vi "Read Sweep Configuration File.vi"(8 "error in (no error)":errorcluster, 10 "Path":path, 11 "SweepControl in":refnum<class "Sweep Control.lvclass">) -> (0 "error out":errorcluster, 2 "Data":variant, 3 "SweepControl out":refnum<class "Sweep Control.lvclass">)   [LabVIEW 2019, in "Sweep Control.lvclass"]
uses:
  Sweep Control.lvclass
  Typedefs/Enum - Experiments.ctl
  Typedefs/Continuous B Sweep JSON--Cluster.ctl
  Typedefs/Enum - Priority.ctl
  Typedefs/Enum - Action.ctl
  Typedefs/Cluster - ScanControl.ctl
  Typedefs/ScanControl.ctl
  Typedefs/Cluster - ScanParamters.ctl
  Typedefs/ScanParamters.ctl
  Typedefs/Sweep Control JSON--Cluster.ctl
  <userlib>/LevyLab/Transport/Control Experiment/Typedefs/Wiring Description--cluster.ctl
  <userlib>/LevyLab/Transport/Control Experiment/Control Experiment.lvclass
  <userlib>/LevyLab/Transport/Control Experiment/Typedefs/Experiment Description--cluster.ctl
  <userlib>/LevyLab/Transport/Transport/Typedefs/Lockin_Sweep JSON--Cluster.ctl
  <userlib>/LevyLab/Transport/Transport/Transport.lvclass
  <userlib>/LevyLab/Lockin-Multichannel/Instrument.DAQ/Typedefs/REF.Channel--Cluster--Array.ctl
  <userlib>/LevyLab/Lockin-Multichannel/Instrument.DAQ/Instrument.DAQ.lvclass
  <userlib>/LevyLab/Lockin-Multichannel/Instrument.DAQ/Typedefs/AO.Channel--Cluster--Array.ctl
  <userlib>/LevyLab/Transport/Control Experiment/Typedefs/Instruments--cluster.ctl
  <userlib>/LevyLab/Krohn Hite 7008/KH7008/typedefs/Filter--Enum.ctl
  <userlib>/LevyLab/Krohn Hite 7008/KH7008/KH7008.lvlib
  <userlib>/LevyLab/Krohn Hite 7008/KH7008/typedefs/couple--Enum.ctl
  <userlib>/LevyLab/Krohn Hite 7008/KH7008/typedefs/shunt--enum.ctl
  <userlib>/LevyLab/Krohn Hite 7008/KH7008/typedefs/Input--Enum.ctl
  <userlib>/LevyLab/Krohn Hite 7008/KH7008/typedefs/gain--enum.ctl
  <userlib>/LevyLab/Krohn Hite 7008/KH7008/typedefs/channel--numeric.ctl
  <userlib>/LevyLab/Krohn Hite 7008/KH7008/typedefs/channelProperties--Cluster.ctl
  <userlib>/LevyLab/Krohn Hite 7008/KH7008/typedefs/allChannelProperties--Array.ctl
  <userlib>/LevyLab/Lockin-Multichannel/Instrument.DAQ/Typedefs/REF.Channel--Cluster.ctl
  <userlib>/LevyLab/Lockin-Multichannel/Instrument.DAQ/Typedefs/AO.Channel.Function--Enum.ctl
  <userlib>/LevyLab/Lockin-Multichannel/Instrument.DAQ/Typedefs/AO.Channel--Cluster.ctl
  <userlib>/LevyLab/Transport/Control Experiment/Typedefs/Instrument Types--enum.ctl
  88356f33-0b26-47ad-bb5b-a6bd6fb0bfd5.vi
  cc7c3cdd-3319-44b7-ab3c-1b04586ceafc.vi
  36e136b2-e9ff-439f-9429-e3ffdab4ccf7.vi
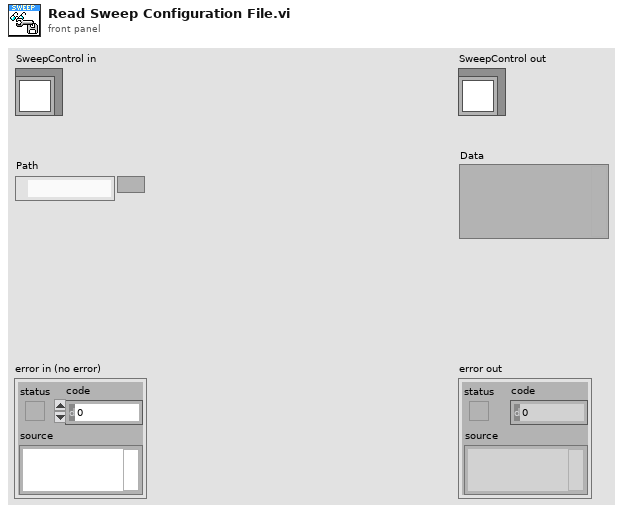
[diagram p1: front panel]
types:
  T1 = typedef "Transport.lvclass/Lockin_Sweep JSON--Cluster.ctl" = cluster{"initialWaitTime":dbl, "sweepTime":dbl, "Return to Start":bool, "sweepChannels":cluster{"Enable?":bool, "Channel":u16, "Start":dbl, "End":dbl, "Pattern":enum16{"Ramp /", "Ramp /\\", "Smooth Ramp _/", "Smooth Ramp _/\\_", "Table"}, "Table":dbl[]}[], "sweepTables":cluster{"Ch":i32, "Table":dbl[]}[]}
  T2 = typedef "Sweep Control.lvclass/Continuous B Sweep JSON--Cluster.ctl" = cluster{"Continuous B Sweep":cluster{"Experiment":T3, "B field values":dbl[]}, "Experiment Description":T4, "Wiring Configuration":T7, "Lockin":cluster{"AOconfig":T8, "REFconfig":T11}, "Krohn Hite":cluster{"Channel Setting":T13}}
  T3 = typedef "Sweep Control.lvclass/Enum - Experiments.ctl" = enum16{"LockinTime", "LockinSweep", "LockinDelayLine"}
  T4 = typedef "Control Experiment.lvclass/Experiment Description--cluster.ctl" = cluster{"User":string, "Device":string, "Device Path":path, "Device Description":string, "Experiment Path":path, "Experiment Description":string, "Instrument":string, "Instruments":T5[], "Sweep":cluster{"key":string, "value":variant}[]}
  T5 = typedef "Control Experiment.lvclass/Instruments--cluster.ctl" = cluster{"class path":path, "Address":string, "Type":T6}
  T6 = typedef "Control Experiment.lvclass/Instrument Types--enum.ctl" = enum16{"DAQ", "Amplifier", "Temperature", "Magnet", "Rotator", "Level", "Capacitance", "Delay Line", "Strain Cell", "VNA", "Source"}
  T7 = typedef "Control Experiment.lvclass/Wiring Description--cluster.ctl" = cluster{"Lockin Ch":i32[], "KH":cluster{"Electrodes":string[], "Labels":string[]}, "not KH":cluster{"Electrodes":string[], "Labels":string[]}}
  T8 = typedef "Instrument.Lockin.lvlib/Instrument.DAQ.lvclass/AO.Channel--Cluster--Array.ctl" = T9[]
  T9 = typedef "Instrument.Lockin.lvlib/Instrument.DAQ.lvclass/AO.Channel--Cluster.ctl" = cluster{"Enable?":bool, "Channel":i32, "Amplitude":dbl, "Offset":dbl, "Frequency":dbl, "Phase":dbl, "Function":T10, "Sweeping?":bool, "Limit AC":bool, "Limit DC?":bool, "Duty Cycle":bool}
  T10 = typedef "Instrument.Lockin.lvlib/Instrument.DAQ.lvclass/AO.Channel.Function--Enum.ctl" = enum16{"sine", "square", "triangle", "saw"}
  T11 = typedef "Instrument.Lockin.lvlib/Instrument.DAQ.lvclass/REF.Channel--Cluster--Array.ctl" = T12[]
  T12 = typedef "Instrument.Lockin.lvlib/Instrument.DAQ.lvclass/REF.Channel--Cluster.ctl" = cluster{"Enable?":bool, "Channel":i32, "Frequency":dbl, "Phase":dbl, "TC":dbl, "Roll-Off":i32}
  T13 = typedef "KH7008.lvlib/allChannelProperties--Array.ctl" = T14[]
  T14 = typedef "KH7008.lvlib/channelProperties--Cluster.ctl" = cluster{"channel":T15, "gain":T16, "input":T17, "shunt":T18, "couple":T19, "filter":T20}
  T15 = typedef "KH7008.lvlib/channel--numeric.ctl" = u16
  T16 = typedef "KH7008.lvlib/gain--enum.ctl" = enum16{"1", "10", "100", "1000"}
  T17 = typedef "KH7008.lvlib/Input--Enum.ctl" = enum16{"OFF", "SE+", "SE-", "DIFF"}
  T18 = typedef "KH7008.lvlib/shunt--enum.ctl" = enum16{"Open", "50", "500", "5k", "50k", "10M"}
  T19 = typedef "KH7008.lvlib/couple--Enum.ctl" = enum16{"AC", "DC"}
  T20 = typedef "KH7008.lvlib/Filter--Enum.ctl" = enum16{"OFF", "ON"}
  T21 = typedef "Sweep Control.lvclass/Sweep Control JSON--Cluster.ctl" = cluster{"Experiment":T3, "Repeat Experiment":i32, "Scan control":T22, "Scan parameters":T26}
  T22 = typedef "Sweep Control.lvclass/ScanControl.ctl" = T23[]
  T23 = typedef "Sweep Control.lvclass/Cluster - ScanControl.ctl" = cluster{"Priority":T24, "Scan name":T25}
  T24 = typedef "Sweep Control.lvclass/Enum - Priority.ctl" = enum16{"Priority 0", "Priority 1", "Priority 2", "Priority 3", "Priority 4", "Priority 5"}
  T25 = typedef "Sweep Control.lvclass/Enum - Action.ctl" = enum16{"OFF", "time", "Lockin Amplitude", "Lockin Frequency", "Lockin Bias", "Delay", "Strain", "DAQ Bias", "Magnet Field", "Temperature", "MW f1", "MW f2", "MW Amplitude1", "MW Amplitude2"}
  T26 = typedef "Sweep Control.lvclass/ScanParamters.ctl" = T27[]
  T27 = typedef "Sweep Control.lvclass/Cluster - ScanParamters.ctl" = cluster{"Start":dbl, "End":dbl, "Step":dbl, "Rate":dbl, "Waveform type":enum16{"linear", "triangle", "power"}, "wait (ms or K)":dbl, "Address":string, "channel":i32}
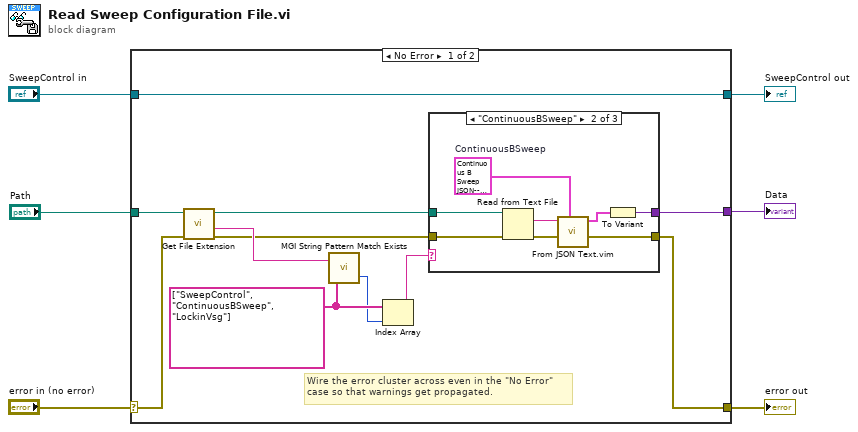
[diagram p0: block diagram]
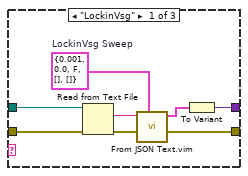
[diagram p2: hidden frame]
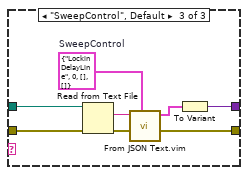
[diagram p3: hidden frame]
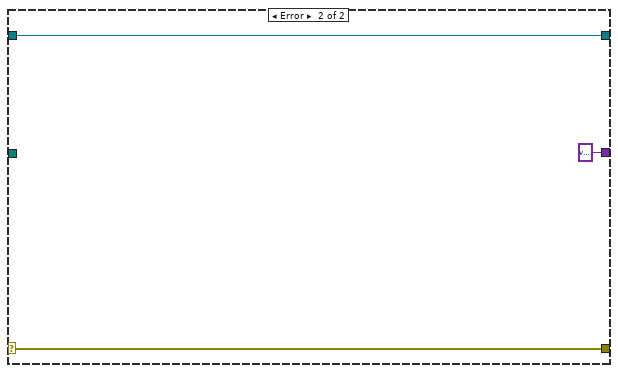
[diagram p4: hidden frame]
diagram:
  n1 = case shown="No Error" "error in (no error)" {
    selector: "error in (no error)" -> [w8 w44]
    tunnel: [w7 w44] -> w5
    tunnel: [w17 w43] -> w3
    tunnel: "SweepControl in" -> [w17 w43]
    tunnel: "Path" -> [w16 _]
    tunnel: [w9 variant ("Variant")] -> w1
    frame No Error {
      w14 = string[] ["SweepControl", "ContinuousBSweep", "LockinVsg"] ("Patterns to Try")
      # "Wire the error cluster across even in the \"No Error\"\ncase so that warnings get propagated."
      n2 = call <vilib>:"Get File Extension.vi"("error in (no error)"=w8, "file"=w16) -> ("error out"=w11:errorcluster, "filename without extension"=w13:string, "dup file"=w10:path)  [unwired: 5 in, 2 out]
      n3 = call <userlib>:"MGI String Pattern Match Exists.vi"("Patterns to Try"=w14, "String"=w13) -> ("Index of First Pattern Matched"=w12:i32)  [unwired: 1 out]
      n4 = Index Array(array=w14, index=w12) -> (element=w15:string)
      n5 = case shown="\"ContinuousBSweep\"" w15 {
        tunnel: w11 -> [w25 w33 w41]
        tunnel: w10 -> [w24 w32 w40]
        tunnel: [w19 w26 w35] -> w9
        tunnel: [w20 w28 w36] -> w7
        frame "LockinVsg" {
          w22 = T1 {"initialWaitTime"=0.001, "sweepTime"=0.0, "Return to Start"=FALSE, "sweepChannels"=[], "sweepTables"=[]}  # LockinVsg Sweep
          n6 = Read from Text File(file (use dialog)=w24, error in=w25) -> (text=w18:string, error out=w21:errorcluster)  [unwired: 2 in, 2 out]
          n7 = call "From JSON Text.vim"("Data Type and Default Value"=w22, "error in (no error)"=w21, "JSON"=w18) -> ("error out"=w20:errorcluster, "Data out"=w23:T1)  [unwired: 7 in]
          n8 = To Variant(anything=w23) -> (Variant=w19:variant)
        }
        frame "ContinuousBSweep" {
          w31 = T2 {"Continuous B Sweep"={"Experiment"=enum."LockinDelayLine", "B field values"=[]}, "Experiment Description"={"User"="", "Device"="", "Device Path"=path "", "Device Description"="", "Experiment Path"=path "", "Experiment Description"="", "Instrument"="", "Instruments"=[], "Sweep"=[]}, "Wiring Configuration"={"Lockin Ch"=[], "KH"={"Electrodes"=[], "Labels"=[]}, "not KH"={"Electrodes"=[], "Labels"=[]}}, "Lockin"={"AOconfig"=[], "REFconfig"=[]}, "Krohn Hite"={"Channel Setting"=[]}}  # ContinuousBSweep
          n9 = Read from Text File(file (use dialog)=w32, error in=w33) -> (text=w30:string, error out=w29:errorcluster)  [unwired: 2 in, 2 out]
          n10 = call "From JSON Text.vim"("Data Type and Default Value"=w31, "error in (no error)"=w29, "JSON"=w30) -> ("error out"=w28:errorcluster, "Data out"=w27:T2)  [unwired: 7 in]
          n11 = To Variant(anything=w27) -> (Variant=w26:variant)
        }
        frame "SweepControl", Default {
          w34 = T21 {"Experiment"=enum."LockinDelayLine", "Repeat Experiment"=0, "Scan control"=[], "Scan parameters"=[]}  # SweepControl
          n12 = Read from Text File(file (use dialog)=w40, error in=w41) -> (text=w38:string, error out=w37:errorcluster)  [unwired: 2 in, 2 out]
          n13 = call "From JSON Text.vim"("Data Type and Default Value"=w34, "error in (no error)"=w37, "JSON"=w38) -> ("error out"=w36:errorcluster, "Data out"=w39:T21)  [unwired: 7 in]
          n14 = To Variant(anything=w39) -> (Variant=w35:variant)
        }
      }
    }
    frame Error {
    }
  }
  "error out" <- w5
  "SweepControl out" <- w3
  "Data" <- w1
